vi "HEWH RLT PRAT.vi"() -> ()   [LabVIEW 2023] (continued)
      frame "Heating_Value_Adjust_LP_UI" {
        n1844 = Variant To Data(error in=w4802, type=0.0, Variant=w4800) -> (data=w4799:dbl, error out=w4801:errorcluster)
        n1845 = call-poly "Enqueue Message.vi"("Priority Message? (F)"=TRUE, "error in (no error)"=w4801, "Message Data"=w4799, "Message"="Heating_Value_Adjust_LP", "Message Queue"=w4796) -> ("error out"=w4798:errorcluster)  [unwired: 5 in, 1 out]
      }
      frame "DisplayValuesFromInficon_LP" {
        # "Update Display - Convert the message data to a string to display in the Data Display indicator."
        n1846 = Variant To Data(error in=w4815, type=T53 {"Gross Heating Value, Vol (Real, Dry)"=0.0, "Nitrogen Component Normalized Mole % (Dry)"=0.0, "Methane Component Normalized Mole % (Dry)"=0.0, "Carbon Dioxide Component Normalized Mole % (Dry)"=0.0, "Ethane Component Normalized Mole % (Dry)"=0.0, "Propane Component Normalized Mole % (Dry)"=0.0, "i-Pentane Component Normalized Mole % (Dry)"=0.0, "i-Butane Component Normalized Mole % (Dry)"=0.0, "n-Butane Component Normalized Mole % (Dry)"=0.0, "n-Pentane Component Normalized Mole % (Dry)"=0.0, "Hexane Component Normalized Mole % (Dry)"=0.0, "Heptane Component Normalized Mole % (Dry)"=0.0, "Gross Wobbe Index, Real(Dry)"=0.0, "Relative Density, Real(Dry)"=0.0, "Propylene Component Normalized Mole % (Dry)"=0.0, "C4 Olefins Component Normalized Mole % (Dry)"=0.0, "Water Component Normalized Mole % (Dry)"=0.0, "Gross Heating Value, Vol (Real, Sat)"=0.0, "Natural Gas Data"=[], "Propane Data"=[]} ("Inficon Data Input"), Variant=w4814) -> (data=w4810:T53, error out=w4808:errorcluster)
        n1847 = Bundle By Name(cluster=w4812, "Inficon Data LP"=w4810) -> (w4811:T67)
        n1848 = call-poly "Enqueue Message.vi"("error in (no error)"=w4808, "Message"="Process_Data", "Message Queue"=w4806) -> ("error out"=w4807:errorcluster)  [unwired: 7 in, 1 out]
        n1849 = Merge Errors(w4807) -> (w4816:errorcluster)
      }
      frame "---------- Vesta ----------" {
        # "Initialize - All initialization work should take place in this message, since other loops can potentially enqueue messages that execute immediately after this one."
      }
      frame "Set_Vesta_VISA_Name_UI" {
        n1850 = Variant To Data(error in=w4825, type="", Variant=w4823) -> (data=w4819:string, error out=w4824:errorcluster)
        n1851 = call-poly "Enqueue Message.vi"("Priority Message? (F)"=TRUE, "error in (no error)"=w4824, "Message Data"=w4819, "Message"="Set_Vesta_VISA_Name", "Message Queue"=w4821) -> ("error out"=w4822:errorcluster)  [unwired: 5 in, 1 out]
      }
      frame "PUT_Vesta_Temp_UI" {
        n1852 = Variant To Data(error in=w4835, type=T44 {"Water Heater Temp (°F)"=0, "Differential  (°F)"=0.0} ("Temperature Parameters"), Variant=w4833) -> (data=w4832:T44, error out=w4834:errorcluster)
        n1853 = call-poly "Enqueue Message.vi"("Priority Message? (F)"=TRUE, "error in (no error)"=w4834, "Message Data"=w4832, "Message"="PUT_Vesta_Temp", "Message Queue"=w4829) -> ("error out"=w4831:errorcluster)  [unwired: 5 in, 1 out]
      }
      frame "DisplayValuesFromVesta" {
        # "Update Display - Convert the message data to a string to display in the Data Display indicator."
        n1854 = Variant To Data(error in=w4848, type=T66 {"Temp_W_Raw_U"=0, "Temp_W_Raw_L"=0, "Temperature Water (F)"=129.1, "Temperature Water Compensated (F)"=133.9, "Temperature Ambient (F)"=74.3, "Setpoint Location (F)"=139.0, "Heat Request"="1F1F", "Fault Ram"="", "PWM DCDC Value"=0, "Pilot Voltage (mV)"=531.5625, "Setpoint Actual (F)"=139.0, "Differential Actual (F)"=10.0, "Setpoint User (F)"=139.0, "Differential User (F)"=10.0, "Termperature FIltered -TCO (F)"=139.0, "Temp_C_Raw_1 - Sensor Voltage"="", "Temp_C_Raw_2 - Sensor Voltage"="", "Chamber Sensor Temperature (F)"=246.0, "LDO Base Temperature (F)"=3276.7, "LDO Timer (sec)"=423, "Disabled (0)"=FALSE, "Warming (1)"=TRUE, "Heating (2)"=FALSE, "Cooling Data Write (3)"=FALSE, "Cooling (4)"=FALSE, "Data Read (5)"=FALSE, "N/A"=FALSE, "Temperature Trip (7)"=FALSE, "Burner"=TRUE} ("Vesta Data Output 2"), Variant=w4847) -> (data=w4839:T66, error out=w4843:errorcluster)
        n1855 = Bundle By Name(cluster=w4846, "Vesta Data Output"=w4839) -> (w4845:T67)
        n1856 = call-poly "Enqueue Message.vi"("error in (no error)"=w4843, "Message"="Process_Data", "Message Queue"=w4841) -> ("error out"=w4842:errorcluster)  [unwired: 7 in, 1 out]
        n1857 = Merge Errors(w4842) -> (w4849:errorcluster)
      }
      frame "---------- Enviracom ----------" {
        # "Initialize - All initialization work should take place in this message, since other loops can potentially enqueue messages that execute immediately after this one."
      }
      frame "Set_Envira_VISA_Name_UI" {
        n1858 = Variant To Data(error in=w4858, type="", Variant=w4856) -> (data=w4855:string, error out=w4857:errorcluster)
        n1859 = call-poly "Enqueue Message.vi"("Priority Message? (F)"=TRUE, "error in (no error)"=w4857, "Message Data"=w4855, "Message"="Set_Envira_VISA_Name", "Message Queue"=w4853) -> ("error out"=w4854:errorcluster)  [unwired: 5 in, 1 out]
      }
      frame "PUT_EnviraCom_Temp_UI" {
        n1860 = Variant To Data(error in=w4868, type=FALSE, Variant=w4866) -> (data=w4865:bool, error out=w4867:errorcluster)
        n1861 = call-poly "Enqueue Message.vi"("Priority Message? (F)"=TRUE, "error in (no error)"=w4867, "Message Data"=w4865, "Message"="PUT_EnviraCom_Temp", "Message Queue"=w4862) -> ("error out"=w4864:errorcluster)  [unwired: 5 in, 1 out]
      }
      frame "---------- Heise Control ----------" {
        # "Place holder, only for organization and readability"
        # "Initialize - All initialization work should take place in this message, since other loops can potentially enqueue messages that execute immediately after this one."
      }
      frame "Set_Heise_VISA_Name_UI" {
        n1862 = Variant To Data(error in=w4880, type="", Variant=w4878) -> (data=w4875:string, error out=w4879:errorcluster)
        n1863 = call-poly "Enqueue Message.vi"("Priority Message? (F)"=TRUE, "error in (no error)"=w4879, "Message Data"=w4875, "Message"="Set_Heise_VISA_Name", "Message Queue"=w4874) -> ("error out"=w4877:errorcluster)  [unwired: 5 in, 1 out]
      }
      frame "DisplayValuesFromHeise" {
        # "Update Display - Convert the message data to a string to display in the Data Display indicator."
        n1864 = Variant To Data(error in=w4893, type=0.0, Variant=w4892) -> (data=w4888:dbl, error out=w4886:errorcluster)
        n1865 = Bundle By Name(cluster=w4890, "Heise Data"=w4888) -> (w4889:T67)
        n1866 = call-poly "Enqueue Message.vi"("error in (no error)"=w4886, "Message"="Process_Data", "Message Queue"=w4884) -> ("error out"=w4885:errorcluster)  [unwired: 7 in, 1 out]
        n1867 = Merge Errors(w4885) -> (w4894:errorcluster)
      }
      frame "---------- Viasala Control ----------" {
        # "Place holder, only for organization and readability"
        # "Initialize - All initialization work should take place in this message, since other loops can potentially enqueue messages that execute immediately after this one."
      }
      frame "Set_Viasala_IP_Name_UI" {
        n1868 = Variant To Data(error in=w4903, type="", Variant=w4901) -> (data=w4898:string, error out=w4902:errorcluster)
        n1869 = call-poly "Enqueue Message.vi"("Priority Message? (F)"=TRUE, "error in (no error)"=w4902, "Message Data"=w4898, "Message"="Set_Viasala_IP_Name", "Message Queue"=w4897) -> ("error out"=w4900:errorcluster)  [unwired: 5 in, 1 out]
      }
      frame "Set_Scan_Rate_UI" {
        n1870 = call-poly "Enqueue Message.vi"("Priority Message? (F)"=TRUE, "error in (no error)"=w4909, "Message Data"="Sample Rate (mS)", "Message"="Set_Scan_Rate", "Message Queue"=w4907) -> ("error out"=w4912:errorcluster)  [unwired: 5 in, 1 out]
        n1871 = Merge Errors(w4912) -> (w4913:errorcluster)
      }
      frame "DisplayValuesFromViasala" {
        # "Update Display - Convert the message data to a string to display in the Data Display indicator."
        n1872 = Variant To Data(error in=w4924, type=T70 {"Temperature Probe 1"=0.0, "Humidity Probe 1"=0.0, "Temperature Probe 2"=0.0, "Humidity Probe 2"=0.0} ("Viasala Data Output"), Variant=w4923) -> (data=w4919:T70, error out=w4917:errorcluster)
        n1873 = Bundle By Name(cluster=w4921, "Viasala Data Output"=w4919) -> (w4920:T67)
        n1874 = call-poly "Enqueue Message.vi"("error in (no error)"=w4917, "Message"="Process_Data", "Message Queue"=w4915) -> ("error out"=w4916:errorcluster)  [unwired: 7 in, 1 out]
        n1875 = Merge Errors(w4916) -> (w4925:errorcluster)
      }
      frame "---------- Agilent Control ----------" {
        # "Place holder, only for organization and readability"
        # "Initialize - All initialization work should take place in this message, since other loops can potentially enqueue messages that execute immediately after this one."
      }
      frame "Set_Agilent_VISA_Name_UI" {
        n1876 = Variant To Data(error in=w4934, type="", Variant=w4932) -> (data=w4929:string, error out=w4933:errorcluster)
        n1877 = call-poly "Enqueue Message.vi"("Priority Message? (F)"=TRUE, "error in (no error)"=w4933, "Message Data"=w4929, "Message"="Set_Agilent_VISA_Name", "Message Queue"=w4928) -> ("error out"=w4931:errorcluster)  [unwired: 5 in, 1 out]
      }
      frame "Set_Agilent_Station_UI" {
        n1878 = Variant To Data(error in=w4944, type=HEWH_Full_Station_IDs."Default" ("Full Station ID"), Variant=w4942) -> (data=w4940:T50, error out=w4943:errorcluster)
        n1879 = call-poly "Enqueue Message.vi"("Priority Message? (F)"=TRUE, "error in (no error)"=w4943, "Message Data"=w4940, "Message"="Set_Agilent_Station", "Message Queue"=w4938) -> ("error out"=w4941:errorcluster)  [unwired: 5 in, 1 out]
      }
      frame "DisplayValuesFromAgilent" {
        # "Update Display - Convert the message data to a string to display in the Data Display indicator."
        n1880 = Variant To Data(error in=w4957, type=T75 {"Location 11 (Channel 111)"=0.0, "Location 12 (Channel 112)"=0.0, "Location 13 (Channel 113)"=0.0, "Location 14 (Channel 114)"=0.0, "Location 15 (Channel 115)"=0.0, "Location 16 (Channel 116)"=0.0, "Location 17 (Channel 109)"=0.0, "Location 18 (Channel 110)"=0.0, "Location 19 (Channel 201)"=0.0, "Location 20 (Channel 202)"=0.0, "Location 21 (Channel 203)"=0.0, "Location 22 (Channel 204)"=0.0, "Location 23 (Channel 205)"=0.0, "Location 24 (Channel 206)"=0.0, "Location 25 (Channel 207)"=0.0, "Location 26 (Channel 208)"=0.0, "Location 27 (Channel 209)"=0.0, "Location 28 (Channel 210)"=0.0, "Location 29 (Channel 211)"=0.0, "Location 30 (Channel 212)"=0.0, "Location 31 (Channel 213)"=0.0, "Location 32 (Channel 214)"=0.0, "Location 33 (Channel 215)"=0.0, "Location 34 (Channel 216)"=0.0, "Location 35 (Channel 107)"=0.0, "Location 36 (Channel 108)"=0.0, "Location 37 (Channel 301)"=0.0, "Location 38 (Channel 302)"=0.0, "Location 39 (Channel 303)"=0.0, "Location 40 (Channel 304)"=0.0, "Location 41 (Channel 305)"=0.0, "Location 42 (Channel 306)"=0.0, "Location 43 (Channel 307)"=0.0, "Location 44 (Channel 308)"=0.0, "Location 45 (Channel 309)"=0.0, "Location 46 (Channel 310)"=0.0, "Location 47 (Channel 311)"=0.0, "Location 48 (Channel 312)"=0.0, "Location 49 (Channel 313)"=0.0, "Location 50 (Channel 314)"=0.0, "Location 51 (Channel 315)"=0.0, "Location 52 (Channel 316)"=0.0, "Location 53 (Channel 105)"=0.0, "Location 54 (Channel 106)"=0.0} ("Agilent Data"), Variant=w4956) -> (data=w4952:T75, error out=w4950:errorcluster)
        n1881 = Bundle By Name(cluster=w4954, "Agilent Data"=w4952) -> (w4953:T67)
        n1882 = call-poly "Enqueue Message.vi"("error in (no error)"=w4950, "Message"="Process_Data", "Message Queue"=w4948) -> ("error out"=w4949:errorcluster)  [unwired: 7 in, 1 out]
        n1883 = Merge Errors(w4949) -> (w4958:errorcluster)
      }
    }
    n1884 = case shown="True" "Enable Arrays" {
      tunnel: w3932 -> [w3945 w3948]
      tunnel: [w3945 w3947] -> w3931
      tunnel: w3930 -> [_ w3946]
      frame False {
      }
      frame True {
        n1885 = Build Array (concatenate)(w3948, w3946) -> (w3947:string[])
        "Main Array" <- w3947
      }
    }
    n1886 = call "Tenney Error Handler - Message Handling Loop.vi"("error in (no error)"=w3934, "Message Queue"=w3936) -> ("dup error in"=w3935:errorcluster)  [unwired: 8 in, 1 out]
  }
  n1887 = disable-structure shown="Enabled" {
    disable-tunnel: [_ TRUE ("Enable Arrays")] -> w2
    frame Disabled {
      n1888 = local read "Enable Arrays"() -> ()  [unwired: 1 out]
    }
    frame Enabled {
    }
  }
  n1889 = control-ref of="Viasala Loop Counter"() -> (w9:refnum<vi>)
  n1890 = control-ref of="Connect Viasala Counter"() -> (w11:refnum<vi>)
  n1891 = control-ref of="Viasala Array"() -> (w8:refnum<vi>)
  n1892 = local read "Enable Arrays"() -> (w12:bool)
  n1893 = control-ref of="Tenney Chamber Loop Counter"() -> (w15:refnum<vi>)
  n1894 = control-ref of="Elapsed Time (Min)"() -> (w16:refnum<vi>)
  n1895 = control-ref of="Connect Tenney Counter"() -> (w17:refnum<vi>)
  n1896 = control-ref of="Tenney Array"() -> (w13:refnum<vi>)
  n1897 = control-ref of="Data Array"() -> (w14:refnum<vi>)
  n1898 = control-ref of="Connection Status Envira"() -> (w4:refnum<vi>)
  n1899 = control-ref of="Connection Status Vesta"() -> (w3:refnum<vi>)
  n1900 = call "Tenney_Main_Temperature_Changer.vi"("Message Queues out"=w32, "Elapsed Time (min) Ref"=w16, "Loop Count Ref"=w15, "Enable Arrays"=w12, "Tenney Array"=w13, "error in"=w31, "Connect Tenney Ref"=w17, "Data Array"=w14) -> ("error out"=w71:errorcluster)  [unwired: 7 in]
  n1901 = call "Tenney_Read_Viasala_Humidity.vi"("Message Queues out"=w32, "Enable Averaging"=TRUE, "Enable Arrays"=w2, "Loop Count Ref"=w9, "error in"=w31, "Connect Viasala Ref"=w11, "Viasala Array"=w8) -> ("error out"=w75:errorcluster)  [unwired: 8 in]
  n1902 = call "HEWH_Alicat_GasMeter.vi"("error in"=w31, "Message Queues out"=w32) -> ("error out"=w56:errorcluster)  [unwired: 9 in]
  n1903 = call "HEWH_Inficon.vi"("error in"=w31, "Message Queues out"=w32) -> ("error out"=w54:errorcluster)  [unwired: 9 in]
  n1904 = call "HEWH_Inficon_LP.vi"("error in"=w31, "Message Queues out"=w32) -> ("error out"=w50:errorcluster)  [unwired: 9 in]
  n1905 = call "HEWH_Ultramat_23.vi"("error in"=w31, "Message Queues out"=w32) -> ("error out"=w53:errorcluster)  [unwired: 9 in]
  n1906 = call "HEWH_Ritter_GasMeter.vi"("error in"=w31, "Debug"=FALSE, "Message Queues out"=w32) -> ("error out"=w52:errorcluster)  [unwired: 8 in]
  n1907 = call "HEWH_HeiseBarometer.vi"("error in"=w31, "Message Queues out"=w32) -> ("error out"=w51:errorcluster)  [unwired: 9 in]
  n1908 = call "HEWH_Emerson_WaterFlowMeter.vi"("error in"=w31, "Message Queues out"=w32) -> ("error out"=w47:errorcluster)  [unwired: 9 in]
  n1909 = call "HEWH_Laurel_WaterFlowMeter.vi"("error in"=w31, "Message Queues out"=w32) -> ("error out"=w46:errorcluster)  [unwired: 9 in]
  n1910 = call "HEWH_WT300.vi"("Manual Range (20 <10> A)"="Manual Range (20 <10> A)", "Range Configuration (True)"="Range Configuration (True)", "error in"=w31, "Enable Auto Range (F: Disable)"="Enable Auto Range (F: Disable)", "Message Queues out"=w32) -> ("error out"=w44:errorcluster)  [unwired: 6 in]
  n1911 = call "HEWH_Agilent_34972A.vi"("error in"=w31, "Message Queues out"=w32) -> ("error out"=w42:errorcluster)  [unwired: 9 in]
  n1912 = call "HEWH GEA3.vi"("error in"=w31, "Message Queues out"=w32) -> ("error out"=w41:errorcluster)  [unwired: 9 in]
  n1913 = call "HEWH GEA3_StationB.vi"("error in"=w31, "Message Queues out"=w32) -> ("error out"=w39:errorcluster)  [unwired: 9 in]
  n1914 = call "HEWH GEA3_StationC.vi"("error in"=w31, "Message Queues out"=w32) -> ("error out"=w38:errorcluster)  [unwired: 9 in]
  n1915 = call "HEWH GEA3_StationD.vi"("error in"=w31, "Message Queues out"=w32) -> ("error out"=w37:errorcluster)  [unwired: 9 in]
  n1916 = call "HEWH MW100.vi"("error in"=w31, "Message Queues out"=w32) -> ("error out"=w36:errorcluster)  [unwired: 9 in]
  n1917 = call "HEWH_EnviraCom_Main.vi"("Envira is working"=w4, "error in"=w31, "Message Queues out"=w32) -> ("error out"=w34:errorcluster)  [unwired: 8 in]
  n1918 = call "HEWH_VESTA_Main.vi"("Vesta is working"=w3, "error in"=w31, "Message Queues out"=w32) -> ("error out"=w33:errorcluster)  [unwired: 8 in]
  n1919 = call "HEWH_Elapsed Timer.vi"("error in"=w31, "Message Queues out"=w32) -> ("error out"=w30:errorcluster)  [unwired: 9 in]
  n1920 = Unregister For Events(event registration refnum=w63, error in=w66) -> (error out=w62:errorcluster)
  n1921 = Merge Errors(w62, w58, w71, w75, w56, w54, w50, w53, w52, w51, w47, w46, w44, w42, w41, w39, w38, w37, w36, w34, w33, w30) -> (w61:errorcluster)
  n1922 = call "Destroy User Event - Stop.vi"("error in (no error)"=w61, "User Event - Stop"=w68) -> ("error out"=w65:errorcluster)  [unwired: 9 in]
  n1923 = disable-structure shown="RUN_TIME_ENGINE==True" {
    disable-tunnel: w65 -> [_ _]
    frame condition #0 (active) {
    }
    frame condition #1 {
      # "Call Quit LabVIEW if running as a built application."
      n1924 = Quit LabVIEW() -> ()  [unwired: 1 in]
    }
  }
  n1925 = disable-structure shown="Disabled" {
    frame Disabled {
      w4961 = i16 2 ("precision (6)")
      w4960 = TRUE ("Add Software Elapsed Time")
      # "There was a reset\ntimer button herer"
      n1926 = call "UTILITY Elapsed Time.vi"() -> ("error out"=w4970:errorcluster, "Main Loop Rate"=→"DAQ Loop Rate":dbl, "Elapsed Time"=w4971:dbl)  [unwired: 7 in, 2 out]
      "Software Elapsed Time" <- w4971
      n1927 = String Length() -> (length=w4972:i32)  [unwired: 1 in]
      n1928 = Greater Than 0?(x=w4972) -> (x > 0?=w4973:bool)
      n1929 = case shown="True" w4973 {
        tunnel: _ -> [w4975 w4990]
        tunnel: [w4975 w4984] -> _
        tunnel: _ -> [_ w4989]
        tunnel: _ -> [_ w4977]
        tunnel: [w4974 w4981] -> _
        tunnel: [w4974 w4980] -> _
        tunnel: [w4974 w4979] -> _
        tunnel: [w4974 w4978] -> _
        tunnel: _ -> [_ w4976]
        frame False {
          w4974 = string[][] [] ("Data (Label,Data)")
        }
        frame True {
          n1930 = call "HEWH Get Agilent Data.vi"("RLT Station Channels"=w4977, "error in (no error)"=w4990, "Test Fixture Hardware"=w4989) -> ("error out"=w4988:errorcluster, "Agilent Calibrated Cluster Array"=w4987:T58[])  [unwired: 5 in, 2 out]
          n1931 = call "HEWH RLT Compile TCs For Station.vi"("Error In"=w4988, "Station ID"="A", "Agilent Cluster Array In"=w4987, "RLT Station Channels In"=w4977) -> ("Error Out"=w4985:errorcluster, "Agilent Cluster Array Out"=w4982:T58[], "RLT Station Channels Out"=w4983:T54, "Data (Label,Data)"=w4981:string[][])  [unwired: 4 in]
          n1932 = case shown="\"PRAT\", \"HEWH RLT\"" w4976 {
            tunnel: w4985 -> [w4992 w5008]
            tunnel: [w4992 w5005] -> w4984
            tunnel: w4983 -> [_ w5004]
            tunnel: w4982 -> [_ w5003]
            tunnel: [w4991 w4995] -> w4980
            tunnel: [w4991 w4994] -> w4979
            tunnel: [w4991 w4993] -> w4978
            frame Default {
              w4991 = string[][] [] ("Data (Label,Data)")
            }
            frame "PRAT", "HEWH RLT" {
              n1933 = call "HEWH RLT Compile TCs For Station.vi"("Error In"=w5008, "Station ID"="B", "Agilent Cluster Array In"=w5003, "RLT Station Channels In"=w5004) -> ("Error Out"=w5007:errorcluster, "Agilent Cluster Array Out"=w5001:T58[], "RLT Station Channels Out"=w5002:T54, "Data (Label,Data)"=w4995:string[][])  [unwired: 4 in]
              n1934 = call "HEWH RLT Compile TCs For Station.vi"("Error In"=w5007, "Station ID"="C", "Agilent Cluster Array In"=w5001, "RLT Station Channels In"=w5002) -> ("Error Out"=w5006:errorcluster, "Agilent Cluster Array Out"=w4999:T58[], "RLT Station Channels Out"=w5000:T54, "Data (Label,Data)"=w4994:string[][])  [unwired: 4 in]
              n1935 = call "HEWH RLT Compile TCs For Station.vi"("Error In"=w5006, "Station ID"="D", "Agilent Cluster Array In"=w4999, "RLT Station Channels In"=w5000) -> ("Error Out"=w5005:errorcluster, "Data (Label,Data)"=w4993:string[][])  [unwired: 4 in, 2 out]
            }
          }
        }
      }
      n1936 = local read "A Timer"() -> (w4963:dbl)
      n1937 = local read "B Timer"() -> (w4965:dbl)
      n1938 = call "UTILITY Elapsed Time General Info.vi"("precision (6)"=w4961, "Add Software Elapsed Time"=w4960, "Error In"=w4970, "Software Elapsed Time"=w4971, "Elapsed Time (sec)"=w4963) -> ("Error Out"=w4964:errorcluster)  [unwired: 2 in, 4 out]
      n1939 = local read "C Timer"() -> (w4968:dbl)
      n1940 = call "UTILITY Elapsed Time General Info.vi"("precision (6)"=w4961, "Add Software Elapsed Time"=w4960, "Error In"=w4964, "Software Elapsed Time"=w4971, "Elapsed Time (sec)"=w4965) -> ("Error Out"=w4966:errorcluster)  [unwired: 2 in, 4 out]
      n1941 = call "UTILITY Elapsed Time General Info.vi"("precision (6)"=w4961, "Add Software Elapsed Time"=w4960, "Error In"=w4966, "Software Elapsed Time"=w4971, "Elapsed Time (sec)"=w4968) -> ("Error Out"=w4967:errorcluster)  [unwired: 2 in, 4 out]
      n1942 = local read "D Timer"() -> (w4969:dbl)
      n1943 = call "UTILITY Elapsed Time General Info.vi"("precision (6)"=w4961, "Add Software Elapsed Time"=w4960, "Error In"=w4967, "Software Elapsed Time"=w4971, "Elapsed Time (sec)"=w4969) -> ()  [unwired: 2 in, 5 out]
    }
    frame Enabled {
    }
  }
